vi "Test_Neo.vi"() -> ()   [LabVIEW 2025]
panel:
  in  "Estado":bool
  out "Analog read":u16
  in  "Pin 2":u8=4 min=4 max=40
  in  "Pin":u8=4 min=4 max=40
  in  "stop":bool
  in  "VISA resource name":refnum<visa-resource-name>
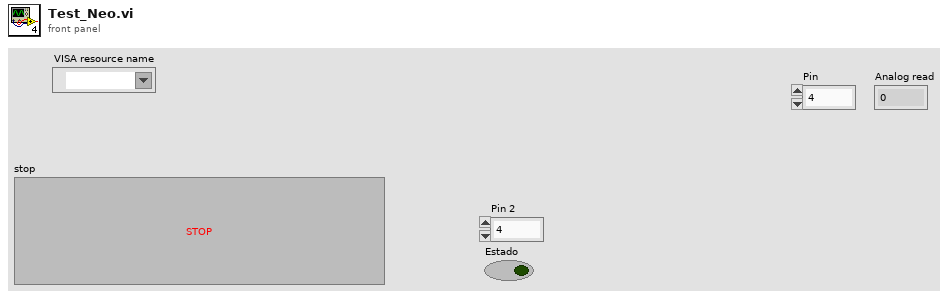
[diagram p1: front panel]
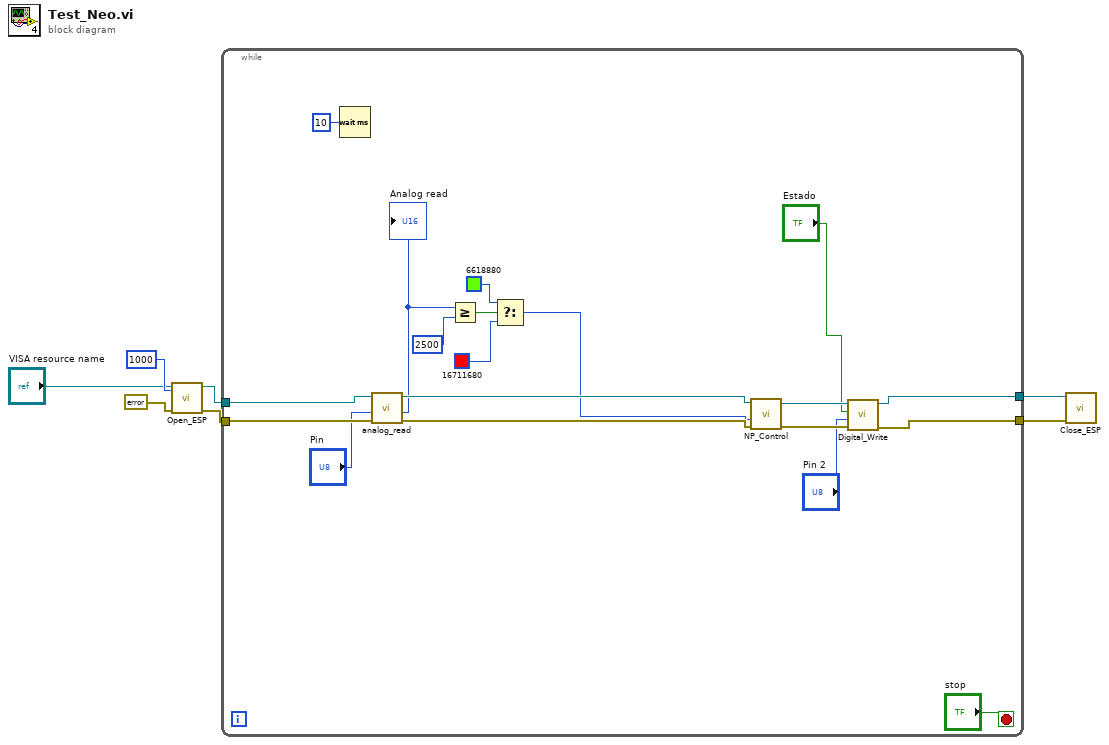
[diagram p0: block diagram]
diagram:
  n1 = call "Open_ESP.vi"("timeout (10sec)"=u32 1000, "error in (no error)"=errorcluster {"status"=FALSE, "code"=0, "source"=""}, "VISA resource name"="VISA resource name") -> ("error out"=w3:errorcluster, "VISA resource name out"=w4:refnum<visa-resource-name>)  [unwired: 7 in]
  n2 = while {
    tunnel: w4 -> [w24]
    tunnel: w3 -> [w21]
    tunnel: [w15] -> w2
    tunnel: [w14] -> w1
    stop <- "stop" stop-if-true
    n3 = Wait (ms)(milliseconds to wait=u32 10) -> ()  [unwired: 1 out]
    n4 = call "analog_read.vi"("error in (no error)"=w21, "Pin"="Pin", "VISA resource name"=w24) -> ("error out"=w22:errorcluster, "Analog read"=w13:u16, "VISA resource name out"=w23:refnum<visa-resource-name>)  [unwired: 5 in, 1 out]
    "Analog read" <- w13
    n5 = Greater Or Equal?(x=w13, y=u16 2500) -> (x >= y?=w11:bool)
    n6 = Select(t=u32 6618880 ("Color Box"), s=w11, f=u32 16711680 ("Color Box")) -> (s? t:f=w8:u32)
    n7 = call "NP_Control.vi"("error in (no error)"=w22, "Color Box"=w8, "VISA resource name"=w23) -> ("error out"=w18:errorcluster, "VISA resource name out"=w19:refnum<visa-resource-name>)  [unwired: 7 in]
    n8 = call "Digital_Write.vi"("error in (no error)"=w18, "Pin"="Pin 2", "Estado"="Estado", "VISA resource name"=w19) -> ("error out"=w14:errorcluster, "VISA resource name out"=w15:refnum<visa-resource-name>)  [unwired: 6 in]
  }
  n9 = call "Close_ESP.vi"("error in (no error)"=w1, "VISA resource name"=w2) -> ()  [unwired: 9 in, 1 out]
